vi "Zero-Pole (DBL Array).vi"(2 "initialize":bool, 3 "dt":dbl=1e-09 min=1e-09 format="%.6f", 4 "gains-zeros-poles":T1(array[cluster]) {"poles" format="%.2f"; "zeros" format="%.2f"; "gain" format="%.2f"}, 5 "input points":dbl[](array[numeric]) format="%.2f") -> (1 "output points":dbl[](array[numeric]) format="%.2f")   [LabVIEW 2017, in "NI_AdvCtrl_continuous linear.lvlib"]
doc: "LabVIEW no longer supports this VI. You can obtain similar functionality by installing the LabVIEW Simulation Module.\n\nCalculates the new output point, where the transfer function and the input point are given. The transfer function is described in gain-zeros-poles notation."
uses:
  <vilib>/addons/control/advanced/NI_AdvCtrl_continuous linear.lvlib
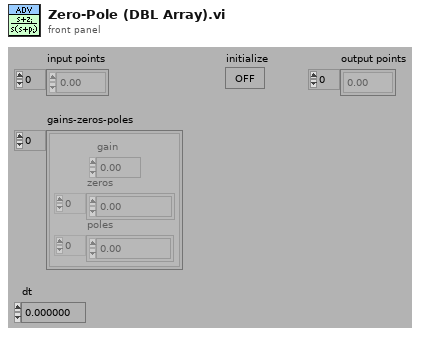
[diagram p1: front panel]
types:
  T1 = cluster{"gain":dbl, "zeros":cdb[], "poles":cdb[]}[]
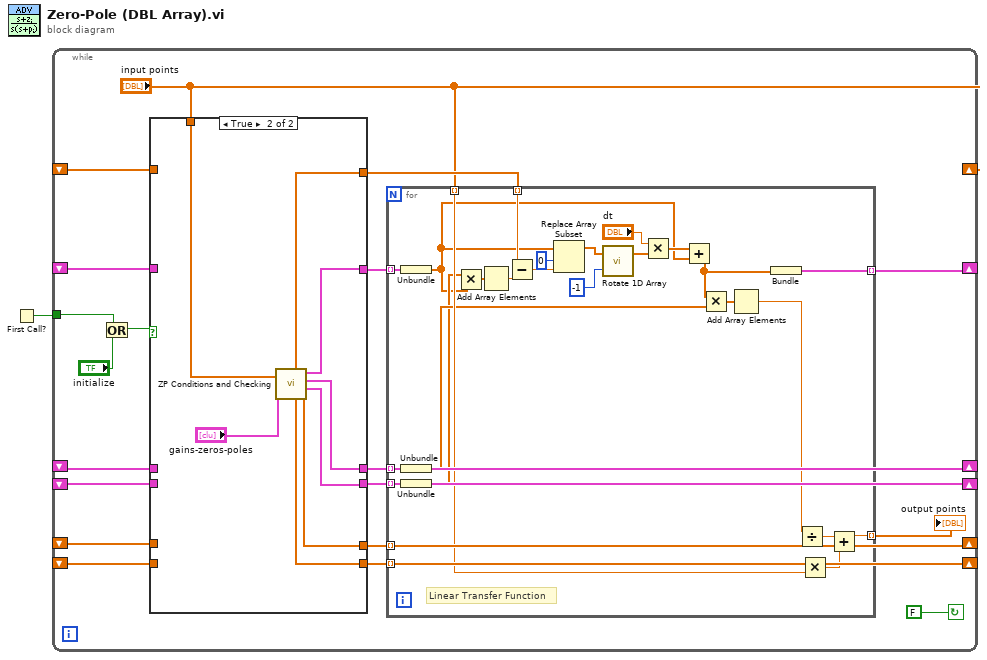
[diagram p0: block diagram]
diagram:
  n1 = First Call?() -> (First Call?: T/F=w1:bool)
  n2 = while {
    shift-left: _ -> [w5]
    shift-right: [w6] -> _
    shift-left: _ -> [w8]
    shift-right: [w10] -> _
    shift-left: _ -> [w13]
    shift-right: ["input points"] -> _
    tunnel: w1 -> [w15]
    shift-left: _ -> [w19]
    shift-right: [w4] -> _
    shift-left: _ -> [w20]
    shift-right: [w18] -> _
    shift-left: _ -> [w9]
    shift-right: [w11] -> _
    stop <- FALSE continue-if-true
    n3 = Or(x=w15, y="initialize") -> (x .or. y?=w3:bool)
    n4 = case shown="True" w3 {
      tunnel: [w51 w53] -> w4
      tunnel: [w52 w56] -> w18
      tunnel: w20 -> [w52 _]
      tunnel: w19 -> [w51 _]
      tunnel: "input points" -> [_ w54]
      tunnel: [w50 w55] -> w14
      tunnel: w13 -> [w50 _]
      tunnel: [w49 w57] -> w11
      tunnel: [w48 w58] -> w10
      tunnel: w9 -> [w49 _]
      tunnel: w8 -> [w48 _]
      tunnel: [w47 w59] -> w7
      tunnel: w5 -> [w47 _]
      frame False {
      }
      frame True {
        n5 = call <vilib>:"ZP Conditions and Checking.vi"("Input Points"=w54, "Zeros-Poles-Gains"="gains-zeros-poles") -> ("previous samples"=w55:dbl[], "additive constants"=w53:dbl[], "internal states"=w59:cluster{dbl[]}[], "numerators"=w57:cluster{"Numerator new":dbl[]}[], "denominators"=w58:cluster{"Denominator new":dbl[]}[], "gains"=w56:dbl[])
      }
    }
    n6 = for {
      tunnel: w4 -> [w46] mode=indexing
      tunnel: w18 -> [w45] mode=indexing
      tunnel: [w34] -> w2 mode=indexing
      tunnel: "input points" -> [w38] mode=indexing
      tunnel: w14 -> [w37] mode=indexing
      tunnel: w11 -> [w32] mode=indexing
      tunnel: w10 -> [w31] mode=indexing
      tunnel: w7 -> [w28] mode=indexing
      tunnel: [w25] -> w6 mode=indexing
      # "Linear Transfer Function"
      n7 = Unbundle(w28) -> (w27:dbl[])
      n8 = Unbundle(w32) -> ("Numerator new"=w30:dbl[])
      n9 = Unbundle(w31) -> ("Denominator new"=w29:dbl[])
      n10 = Multiply(x=w29, y=w27) -> (x*y=w42:dbl[])
      n11 = Add Array Elements(numeric array=w42) -> (sum=w41:dbl)
      n12 = Subtract(x=w37, y=w41) -> (x-y=w44:dbl)
      n13 = Replace Array Subset(array=w27, new element=w44, index=0 ("Index")) -> (w24:dbl[])
      n14 = call <vilib>:"Rotate 1D Array.vi"("n"=-1, "array"=w24) -> ("array (last n elements first)"=w23:dbl[])  [unwired: 1 out]
      n15 = Multiply(x="dt", y=w23) -> (x*y=w40:dbl[])
      n16 = Add(x=w40, y=w27) -> (x+y=w26:dbl[])
      n17 = Multiply(x=w26, y=w30) -> (x*y=w39:dbl[])
      n18 = Add Array Elements(numeric array=w39) -> (sum=w36:dbl)
      n19 = Bundle(w26) -> (w25:cluster{dbl[]})  [unwired: 1 in]
      n20 = Divide(x=w36, y=w45) -> (x/y=w35:dbl)
      n21 = Multiply(x=w46, y=w38) -> (x*y=w33:dbl)
      n22 = Add(x=w35, y=w33) -> (x+y=w34:dbl)
    }
    "output points" <- w2
  }
